vi "WSVCAP SHL Host LL I2C Build Socket Mask.vi"(0 "DUT Mask Array (All)":bool[](array[boolean])=[TRUE, TRUE, TRUE, TRUE, TRUE, TRUE, TRUE, TRUE, TRUE, TRUE, TRUE, TRUE, TRUE, TRUE, TRUE, TRUE, TRUE, TRUE, TRUE, TRUE, TRUE, TRUE, TRUE, TRUE], 7 "DUT Mask Mode (Custom)":T1) -> (4 "Socket Mask Set [U64]":u64 format="%06x")   [LabVIEW 2017]
uses:
  Type Defs/WSVCAP SHL I2C DUT Mask Mode Enum.ctl
panel:
  # "DUT 01"
  # "DUT 02"
  # "DUT 03"
  # "DUT 04"
  # "DUT 05"
  # "DUT 06"
  # "DUT 07"
  # "DUT 08"
  # "DUT 09"
  # "DUT 10"
  # "DUT 11"
  # "DUT 12"
  # "DUT 13"
  # "DUT 14"
  # "DUT 15"
  # "DUT 16"
  # "DUT 17"
  # "DUT 18"
  # "DUT 19"
  # "DUT 20"
  # "DUT 21"
  # "DUT 22"
  # "DUT 23"
  # "DUT 24"
  # "C"
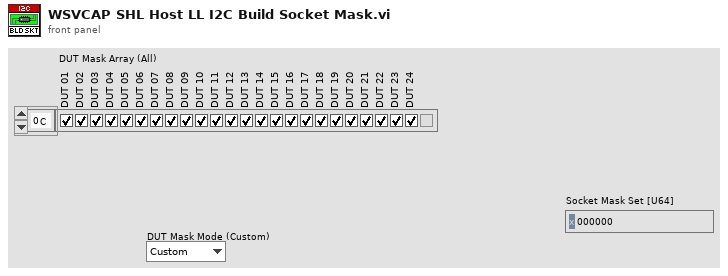
[diagram p1: front panel]
types:
  T1 = typedef "WSVCAP SHL I2C DUT Mask Mode Enum.ctl" = enum16{"Custom", "All"}
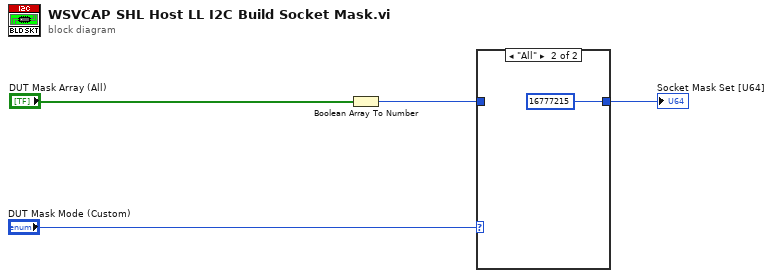
[diagram p0: block diagram]
diagram:
  n1 = Boolean Array To Number(Boolean array="DUT Mask Array (All)") -> (number=w2:u64)
  n2 = case shown="\"All\"" "DUT Mask Mode (Custom)" {
    tunnel: [w5 u64 16777215 ("Socket Mask [U64]")] -> w3
    tunnel: w2 -> [w5 _]
    frame "Custom" {
    }
    frame "All" {
    }
  }
  "Socket Mask Set [U64]" <- w3
